vi "plot_sailing_points.vi"(8 "Intermediate\nWaypoints":refnum<class "Waypoint.lvclass">[](array[class]), 9 "MapDistanceInfo":T1 {"Top Left Pixel UTM"."North" format="%#_10f"; "Top Left Pixel UTM"."East" format="%#_8f"; "Bottom Right Pixel UTM"."North" format="%#_10f"; "Bottom Right Pixel UTM"."East" format="%#_8f"}, 11 "Map in":T3) -> (1 "MapDistanceInfo OUT":T1 {"Top Left Pixel UTM"."North" format="%#_10f"; "Top Left Pixel UTM"."East" format="%#_8f"; "Bottom Right Pixel UTM"."North" format="%#_10f"; "Bottom Right Pixel UTM"."East" format="%#_8f"}, 2 "WP Outside Img":bool, 3 "Map Out":T3)   [LabVIEW 2013]
uses:
  cRIO_Code/Logic/Classes/Waypoint/Waypoint.lvclass
  <vilib>/vision/Image Controls.llb/IMAQ Image.ctl
  TypeDef/map_metadata.ctl
  cRIO_Code/Data/TypeDefs/UTM Location.ctl
panel:
  out "Waypoint Array":refnum<class "Waypoint.lvclass">[](array[class])
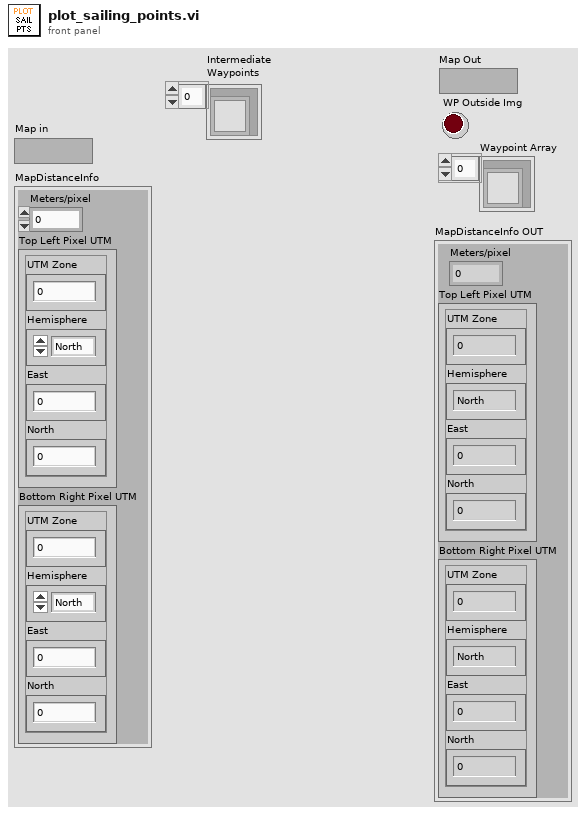
[diagram p1: front panel]
types:
  T1 = typedef "map_metadata.ctl" = cluster{"Meters/pixel":dbl, "Top Left Pixel UTM":T2, "Bottom Right Pixel UTM":T2}
  T2 = typedef "UTM Location.ctl" = cluster{"UTM Zone":dbl, "Hemisphere":enum16{"North", "South"}, "East":dbl, "North":dbl}
  T3 = typedef "IMAQ Image.ctl" = refnum<image>
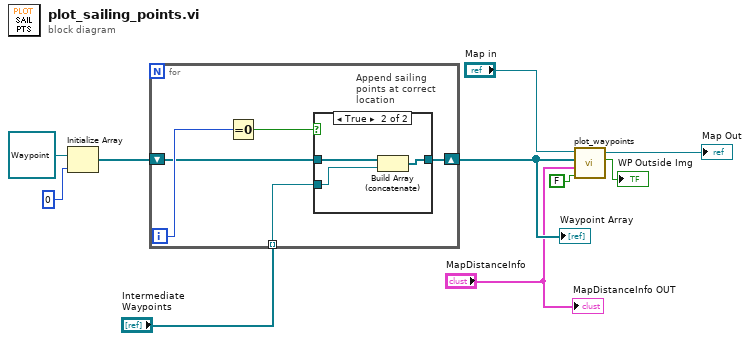
[diagram p0: block diagram]
diagram:
  n1 = Initialize Array "Initialize Array"(refnum<class "Waypoint.lvclass"> refnum ("Waypoint Out"), 0 ("dimension size")) -> (w8:refnum<class "Waypoint.lvclass">[])
  n2 = for {
    shift-right: [w13] -> w7
    shift-left: w8 -> [w12]
    tunnel: "Intermediate\nWaypoints" -> [w11] mode=indexing
    i -> [w15]
    n3 = Equal To 0?(x=w15) -> (x = 0?=w14:bool)
    n4 = case "Append sailing\npoints at correct\nlocation" shown="True" w14 {
      tunnel: w12 -> [w16 w19]
      tunnel: [w16 w18] -> w13
      tunnel: w11 -> [_ w17]
      frame False {
      }
      frame True {
        n5 = Build Array (concatenate)(w19, w17) -> (w18:refnum<class "Waypoint.lvclass">[])
      }
    }
  }
  "Waypoint Array" <- w7
  n6 = call "plot_waypoints.vi"("Mission Waypoint?"=FALSE, "MapDistanceInfo"="MapDistanceInfo", "Waypoint Array"=w7, "Map in"="Map in") -> ("WP Outside Img"=→"WP Outside Img":bool, "Map Out"=→"Map Out":T3)  [unwired: 6 in]
  "MapDistanceInfo OUT" <- "MapDistanceInfo"
